vi "EnableAxis.vi"(4 "error in (no error)":errorcluster, 7 "axis in":cluster{"keyHandle":u32, "nodeId":u16}={"keyHandle"=0, "nodeId"=1}) -> (0 "error out":errorcluster, 3 "axis out":cluster{"keyHandle":u32, "nodeId":u16}={"keyHandle"=0, "nodeId"=1})   [LabVIEW 2017, in "maxonEPOS.lvlib"]
doc: "<B>EnableAxis</B> clears all errors an sets the device to enable state."
uses:
  Examples/maxonEPOS.lvlib
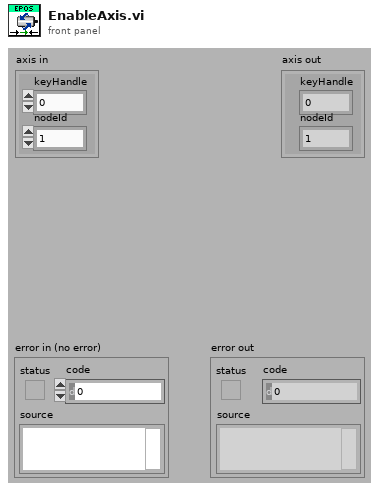
[diagram p1: front panel]
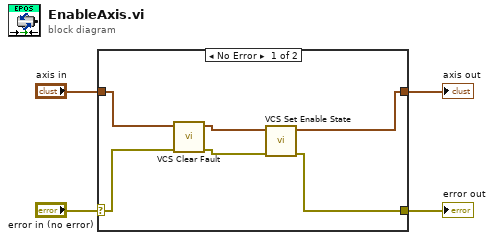
[diagram p0: block diagram]
diagram:
  n1 = case shown="No Error" "error in (no error)" {
    selector: "error in (no error)" -> [w9 w12]
    tunnel: [w7 w12] -> w3
    tunnel: [w6 w11] -> w2
    tunnel: "axis in" -> [w10 w11]
    frame No Error {
      n2 = call "VCS Clear Fault.vi"("error in (no error)"=w9, "axis in"=w10) -> ("error out"=w8:errorcluster, "axis out"=w5:cluster{"keyHandle":u32, "nodeId":u16})  [unwired: 8 in]
      n3 = call "VCS Set Enable State.vi"("error in (no error)"=w8, "axis in"=w5) -> ("error out"=w7:errorcluster, "axis out"=w6:cluster{"keyHandle":u32, "nodeId":u16})  [unwired: 8 in]
    }
    frame Error {
    }
  }
  "error out" <- w3
  "axis out" <- w2
